vi "setUp.vi"(8 "error in (no error)":errorcluster, 11 "reference in":refnum<class "Disabled Custom Device.lvclass">) -> (0 "error out":errorcluster, 3 "reference out":refnum<class "Disabled Custom Device.lvclass">)   [LabVIEW 2020, in "Disabled Custom Device.lvclass"]
doc: "setUp runs prior to the test method during test execution. Use this method to initialize any object data required by your tests."
uses:
  Disabled Custom Device.lvclass
  C:/Program Files (x86)/National Instruments/LabVIEW 2020/vi.lib/addons/_JKI Toolkits/VI Tester/TestCase.llb/TestCase.lvclass
  Disabled Custom Device.lvclass/Disabled Custom Device.ctl
  <vilib>/addons/_JKI Toolkits/VI Tester/TestCase.llb/TestCase.lvclass
  niveristand-custom-device-testing-tools/VeriStandTestUtilities/VeriStandTestUtilities.lvlib
  Scripting/AIM/AIM ARINC 429 Scripting.lvlib
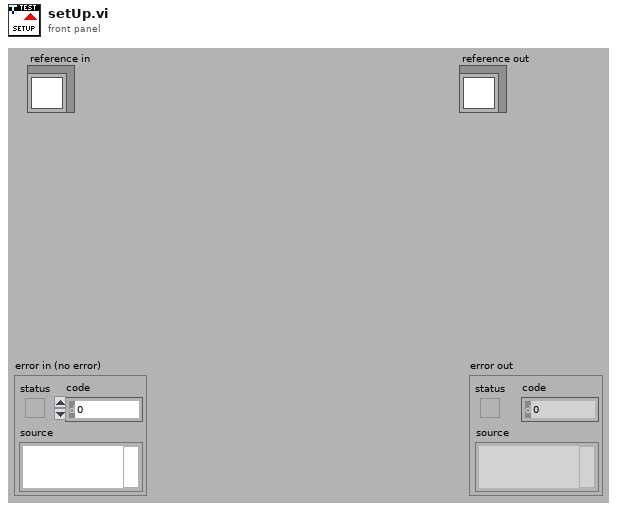
[diagram p1: front panel]
types:
  T1 = typedef "Custom Device API.lvlib/Custom Device Item Ref.ctl" = u64
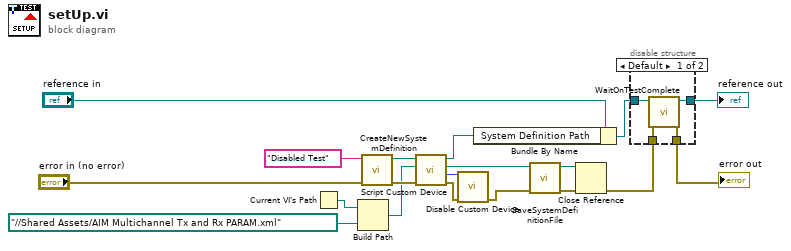
[diagram p0: block diagram]
diagram:
  n1 = Current VI's Path() -> (path=w6:path)
  n2 = Build Path(base path=w6, name or relative path=path "../../Shared Assets/AIM Multichannel Tx and Rx PARAM.xml" ("Hardware File Path")) -> (appended path=w4:path)
  n3 = call "CreateNewSystemDefinition.vi"("error in"="error in (no error)", "System Definition Name"="Disabled Test" ("Channel")) -> ("error out"=w14:errorcluster, "System Definition Path"=w13:path)  [unwired: 8 in]
  n4 = call "Script Custom Device.vi"("error in"=w14, "Parameter File Path"=w4, "System Definition File Path In"=w13) -> ("error out"=w3:errorcluster, "AIM ARINC 429 custom device out"=w2:T1, "System Definition Reference"=w12:refnum<k24>, "System Definition File Path Out"=w5:path)  [unwired: 5 in]
  n5 = call "Disable Custom Device.vi"("error in (no error)"=w3, "AIM ARINC 429 ref"=w2) -> ("error out"=w1:errorcluster)  [unwired: 8 in, 1 out]
  n6 = Bundle By Name(cluster="reference in", "System Definition Path"=w5) -> (w8:refnum<class "Disabled Custom Device.lvclass">)
  n7 = call "SaveSystemDefinitionFile.vi"("error in (no error)"=w1, "System Definition Reference in"=w12) -> ("error out"=w10:errorcluster, "System Definition Reference out"=w9:refnum<k24>)  [unwired: 8 in]
  n8 = Close Reference(reference=w9, error in (no error)=w10) -> (error out=w7:errorcluster)
  n9 = disable-structure shown="Default" {
    disable-tunnel: w7 -> [w23 w24]
    disable-tunnel: [w22 w24] -> w19
    disable-tunnel: [w21 w25] -> w17
    disable-tunnel: w8 -> [w20 w25]
    frame condition #0 (active) {
      n10 = call <vilib>:"WaitOnTestComplete.vi"("error in (no error)"=w23, "TestCase in"=w20) -> ("error out"=w22:errorcluster, "TestCase out"=w21:refnum<class "Disabled Custom Device.lvclass">)  [unwired: 8 in]
    }
    frame condition #1 {
    }
  }
  "error out" <- w19
  "reference out" <- w17
